vi "Get Rotate Data.vi"(8 "error in (no error)":errorcluster, 10 "IND":T1 {"Rotate_IND" items=["стоп", "Качалка Режим Авто", "Качалка Режим Ручной"]; "Termex_IND" items=["Термостат старт"=1, "Термостат стоп"=0]; "Mix_IND" items=["Мешалка движение вперёд"=1, "Мешалка движение назад"=2, "Мешалка стоп"=0]}, 11 "Rotate Ref":refnum<vi>) -> (0 "error out":errorcluster)   [LabVIEW 2023, in "GUI.lvlib" / "gui.lvclass"]
uses:
  gui.lvclass
  gui.lvclass/gui.ctl
  Drive/Rotation Control Type.ctl
  Drive/Drive.lvlib
  Modbus PLC/Modbus PLC/Data.ctl
  Modbus PLC/Modbus PLC/Modbus PLC.lvclass
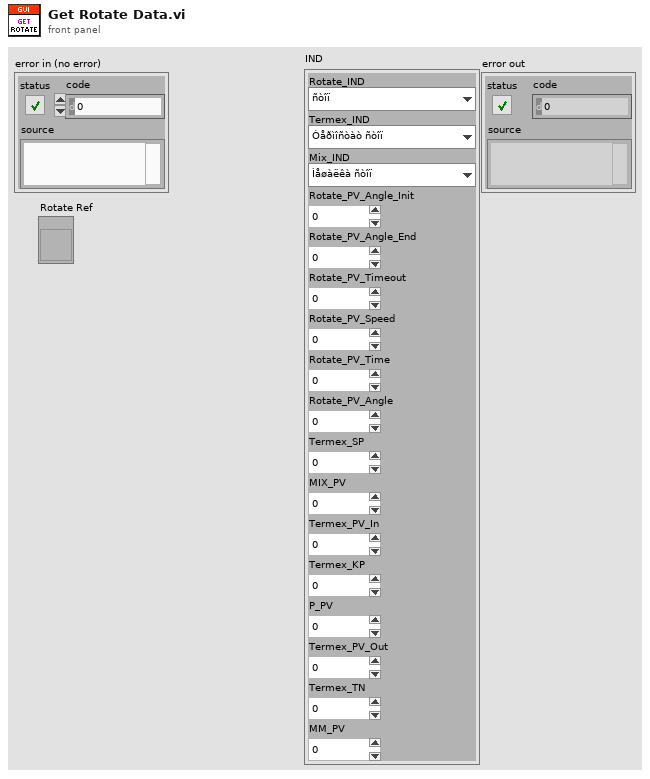
[diagram p1: front panel]
types:
  T1 = typedef "Modbus PLC.lvlib/Modbus PLC.lvclass/Data.ctl" = cluster{"Rotate_IND":u16, "Termex_IND":u16, "Mix_IND":u16, "Rotate_PV_Angle_Init":u16, "Rotate_PV_Angle_End":u16, "Rotate_PV_Timeout":u16, "Rotate_PV_Speed":u16, "Rotate_PV_Time":u16, "Rotate_PV_Angle":u16, "Termex_SP":sgl, "MIX_PV":u16, "Termex_PV_In":sgl, "Termex_KP":sgl, "P_PV":sgl, "Termex_PV_Out":sgl, "Termex_TN":sgl, "MM_PV":sgl}
  T2 = typedef "Drive.lvlib/Rotation Control Type.ctl" = cluster{"Mode":u16, "PV Angle":dbl, "SP_Angle":dbl, "Rotate Angle":dbl, "Timeout":dbl, "Start":bool, "Home":bool}
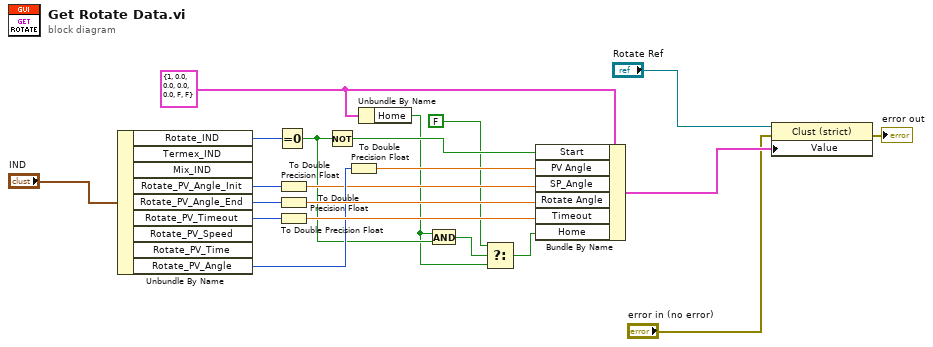
[diagram p0: block diagram]
diagram:
  w8 = T2 {"Mode"=1, "PV Angle"=0.0, "SP_Angle"=0.0, "Rotate Angle"=0.0, "Timeout"=0.0, "Start"=FALSE, "Home"=FALSE} ("Rotate")
  n1 = Unbundle By Name("IND") -> ("Rotate_IND"=w18:u16, "Rotate_PV_Angle_Init"=w10:u16, "Rotate_PV_Angle_End"=w14:u16, "Rotate_PV_Timeout"=w16:u16, "Rotate_PV_Angle"=w12:u16)  [unwired: 4 out]
  n2 = Equal To 0?(x=w18) -> (x = 0?=w7:bool)
  n3 = To Double Precision Float(number=w10) -> (double precision float=w9:dbl)
  n4 = To Double Precision Float(number=w14) -> (double precision float=w13:dbl)
  n5 = To Double Precision Float(number=w16) -> (double precision float=w15:dbl)
  n6 = Not(x=w7) -> (.not. x?=w17:bool)
  n7 = To Double Precision Float(number=w12) -> (double precision float=w11:dbl)
  n8 = Unbundle By Name(w8) -> ("Home"=w5:bool)
  n9 = And(x=w5, y=w7) -> (x .and. y?=w6:bool)
  n10 = Select(t=FALSE, s=w6, f=w5) -> (s? t:f=w3:bool)
  n11 = Bundle By Name(cluster=w8, "Start"=w17, "PV Angle"=w11, "SP_Angle"=w9, "Rotate Angle"=w13, "Timeout"=w15, "Home"=w3) -> (w21:T2)
  n12 = property class="Clust (strict)"(reference="Rotate Ref", error in="error in (no error)", "Value"=w21) -> (error out=→"error out":errorcluster)  [unwired: 1 out]
